vi "Actor Core.vi"(8 "error in":errorcluster, 11 "State in":refnum<class "System.lvclass">) -> (0 "error out":errorcluster, 3 "Actor out":refnum<class "Actor.lvclass">)   [LabVIEW 2013, in "System.lvlib" / "System.lvclass"]
doc: "(<B>Filename</B>: Actor Framework.lvlib:Actor.lvclass:Actor Core.vi)\n\nThis override invokes Entry.vi on the initial state, prior to calling the parent Actor Core. Adding this behavior to Actor Core (instead of an override of Pre Launch Init.vi) allows the initial state to launch a nested actor as part of its entry behavior.\n\nReceives messages to the actor, reacts to them, and initiates any error handling that may shut the actor down.\n\nDescendant classes may override this VI to append parallel tasks for the actor to complete while it handles messages. Overrides use the Call Parent Method node."
uses:
  System.lvclass
  <vilib>/ActorFramework/Actor/Actor.lvclass
  System Status.ctl
  SystemStates.ctl
  Command Processor/Command Processor Status.ctl
  Current Previous State Status.ctl
  State Status.ctl
  Command Processor/Command/Command Status.ctl
  Command Processor/Command/State Status.ctl
  System.lvclass/System.ctl
  <vilib>/ni/Actors/State Actor/State Actor/State Actor.lvclass
  Command Processor/Command Processor.lvclass
  Command Processor/Command/Command.lvclass
panel:
  in  "System Status":T1
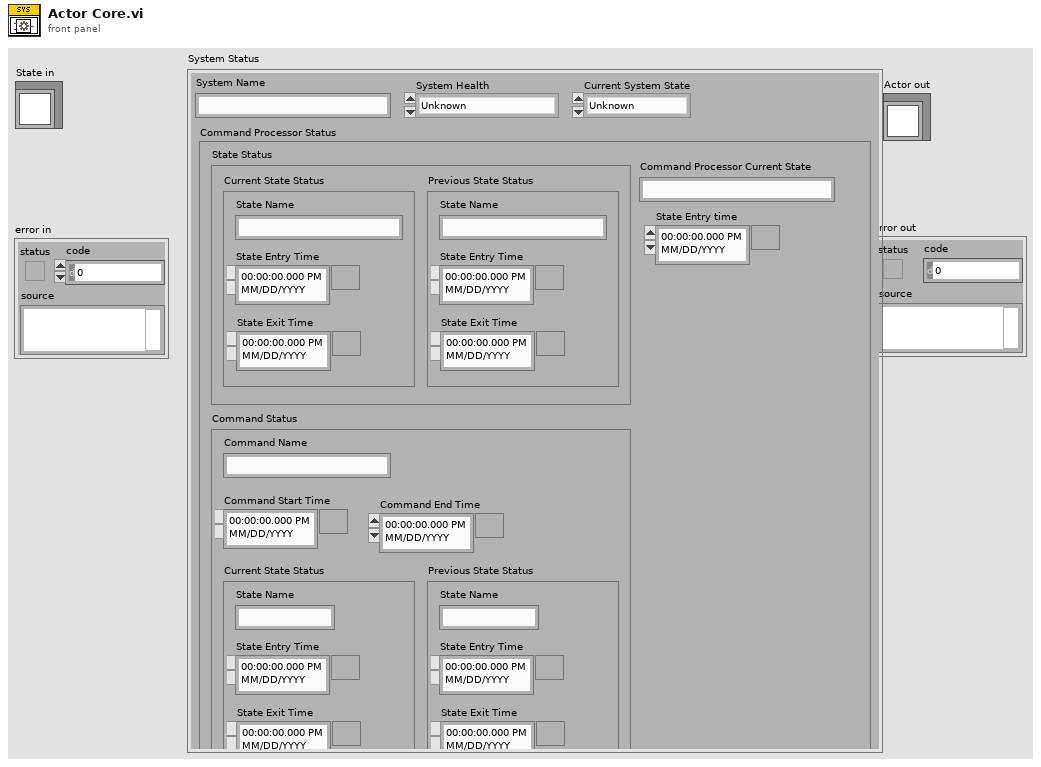
[diagram p1: front panel]
types:
  T1 = typedef "System.lvlib/System.lvclass/System Status.ctl" = cluster{"Current System State":T2, "System Health":enum16{"Unknown", "Good", "Poor", "Bad"}, "System Name":string, "Command Processor Status":T3}
  T2 = typedef "System.lvlib/System.lvclass/SystemStates.ctl" = enum16{"Unknown", "Running", "Stopped"}
  T3 = typedef "Command Processor.lvlib/Command Processor.lvclass/Command Processor Status.ctl" = cluster{"State Entry time":timestamp, "State Status":T4, "Command Processor Current State":string, "Command Status":T6}
  T4 = typedef "Current Previous State Status.ctl" = cluster{"Current State Status":T5, "Previous State Status":T5}
  T5 = typedef "State Status.ctl" = cluster{"State Name":string, "State Entry Time":timestamp, "State Exit Time":timestamp}
  T6 = typedef "Command Processor.lvlib/Command.lvlib/Command.lvclass/Command Status.ctl" = cluster{"Command Name":string, "Current State Status":T7, "Command Start Time":timestamp, "Command End Time":timestamp, "Previous State Status":T7}
  T7 = typedef "Command Processor.lvlib/Command.lvlib/Command.lvclass/State Status.ctl" = cluster{"State Name":string, "State Entry Time":timestamp, "State Exit Time":timestamp}
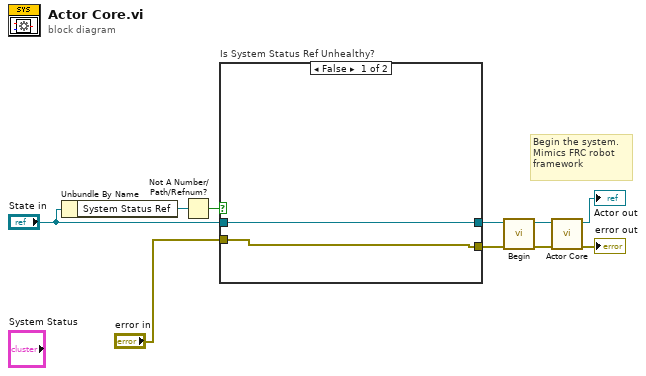
[diagram p0: block diagram]
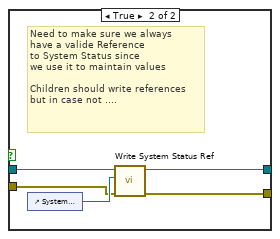
[diagram p2: hidden frame]
diagram:
  # "Begin the system.\nMimics FRC robot \nframework"
  n1 = Unbundle By Name("State in") -> ("System Status Ref"=w7:refnum<vi>)
  n2 = Not A Number/Path/Refnum?(number/path/refnum=w7) -> (NaN/Path/Refnum?=w6:bool)
  n3 = case "Is System Status Ref Unhealthy?" shown="False" w6 {
    tunnel: "State in" -> [w12 w17]
    tunnel: [w12 w15] -> w5
    tunnel: "error in" -> [w11 w14]
    tunnel: [w11 w13] -> w2
    frame False {
    }
    frame True {
      # "Need to make sure we always\nhave a valide Reference\nto System Status since\nwe use it to maintain values\n\nChildren should write references \nbut in case not ...."
      n4 = control-ref of="System Status"() -> (w16:refnum<vi>)
      n5 = call-dynamic "Write System Status Ref.vi"("error in (no error)"=w14, "System Status Ref"=w16, "System in"=w17) -> ("error out"=w13:errorcluster, "System out"=w15:refnum<class "System.lvclass">)  [unwired: 7 in]
    }
  }
  n6 = call-dynamic "Begin.vi"("error in (no error)"=w2, "System in"=w5) -> ("error out"=w1:errorcluster, "System out"=w4:refnum<class "System.lvclass">)  [unwired: 8 in]
  n7 = call-parent "Actor Core.vi"("error in"=w1, "State in"=w4) -> ("error out"=→"error out":errorcluster, "Actor out"=→"Actor out":refnum<class "Actor.lvclass">)  [unwired: 8 in]
